vi "Fluke Molbox 1 Plus Acquire Totalize Cycle Results.vi"(0 "VISA resource name":refnum<visa-resource-name>, 1 "Gas Type (Nitrogen)":u16(ring) items=["Nitrogen", "Helium", "Argon", "Hydrogen", "Oxygen", "Methane", "Ethylene", "Propane", "Ethane", "Butane", "Carbon Monoxide", "Air", "Hexafluoroethane", "Nitrous Oxide", "Carbon Tetrafluoride", "Sulfur Hexafluoride", "Fluoroform", "Carbon Dioxide", "Xenon", "Octofluorocyclobutane"], 5 "Period Hours (0)":i32, 7 "Period Minutes (1)":i32=1, 9 "Period Seconds (0)":i32, 12 "K Factor (1.0)":dbl=1.0) -> (6 "Seconds Elapsed":dbl, 8 "Total Flow":dbl)   [LabVIEW 2023]
doc: "Completes a totalize cycle and returns the total flow that was accumulated in the cycle of which the length is inputted by the user."
uses:
  Fluke Molbox 1 Plus.lvlib
panel:
  in  "Serial Configuration":T1={"Baud Rate"=9600, "Parity"=0, "Data Bits"=7, "Stop Bits"=10} {"Stop Bits" items=["1"=10, "2"=20]; "Data Bits" items=["7"=7, "8"=8]; "Parity" items=["None", "Odd", "Even"]; "Baud Rate" items=["300"=300, "600"=600, "1200"=1200, "2400"=2400, "4800"=4800, "9600"=9600, "19200"=19200]}
  # "(c) 2012 National Instruments.  ALL RIGHTS RESERVED."
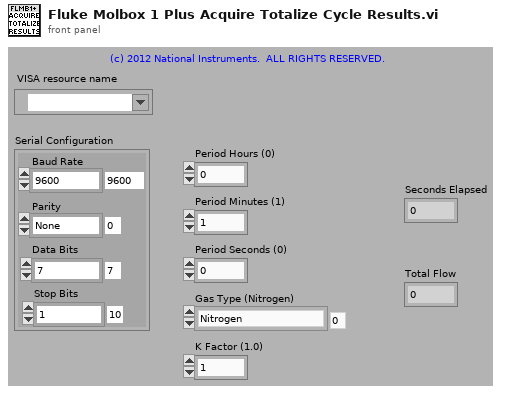
[diagram p1: front panel]
types:
  T1 = cluster{"Baud Rate":u32, "Parity":u16, "Data Bits":u16, "Stop Bits":u16}
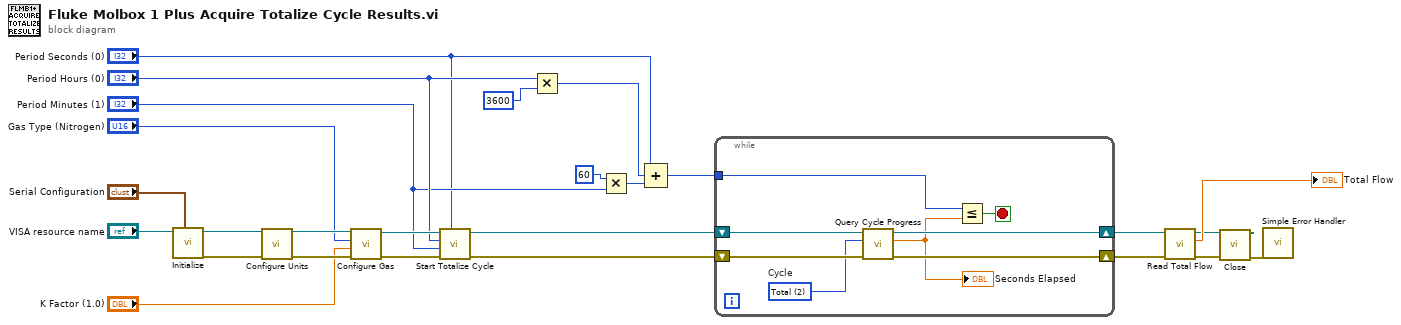
[diagram p0: block diagram]
diagram:
  n1 = call "Initialize.vi"("Serial Configuration"="Serial Configuration", "VISA resource name"="VISA resource name") -> ("error out"=w24:errorcluster, "VISA resource name out"=w25:refnum<visa-resource-name>)  [unwired: 8 in]
  n2 = call "Configure Units.vi"("VISA resource name"=w25, "error in (no error)"=w24) -> ("VISA resource name out"=w21:refnum<visa-resource-name>, "error out"=w20:errorcluster)  [unwired: 12 in]
  n3 = call "Configure Gas.vi"("error in (no error)"=w20, "K Factor (1.0)"="K Factor (1.0)", "Gas Type (0: Nitrogen)"="Gas Type (Nitrogen)", "VISA resource name"=w21) -> ("error out"=w14:errorcluster, "VISA resource name out"=w15:refnum<visa-resource-name>)  [unwired: 6 in]
  n4 = call "Start Totalize Cycle.vi"("Period Seconds (0)"="Period Seconds (0)", "error in (no error)"=w14, "Period Minutes (1)"="Period Minutes (1)", "Period Hours (0)"="Period Hours (0)", "VISA resource name"=w15) -> ("error out"=w16:errorcluster, "VISA resource name out"=w17:refnum<visa-resource-name>)  [unwired: 5 in]
  n5 = Multiply(x="Period Hours (0)", y=u32 3600) -> (x*y=w7:u32)
  n6 = Multiply(x=u32 60, y="Period Minutes (1)") -> (x*y=w8:u32)
  n7 = Compound Arithmetic op=ADD("Period Seconds (0)", w7, w8) -> (w5:u32)
  n8 = while {
    shift-right: [w29] -> w22
    shift-left: w16 -> [w33]
    shift-right: [w30] -> w23
    shift-left: w17 -> [w34]
    tunnel: w5 -> [w28]
    stop <- w32 stop-if-true
    w31 = u16 2 items=["Leak Check", "Purge", "Total"]  # Cycle
    n9 = call "Query Cycle Progress.vi"("error in (no error)"=w33, "Cycle (0: Average Flow)"=w31, "VISA resource name"=w34) -> ("error out"=w29:errorcluster, "Seconds"=w27:dbl, "VISA resource name out"=w30:refnum<visa-resource-name>)  [unwired: 6 in]
    "Seconds Elapsed" <- w27
    n10 = Less Or Equal?(x=w28, y=w27) -> (x <= y?=w32:bool)
  }
  n11 = call "Read Total Flow.vi"("error in (no error)"=w22, "VISA resource name"=w23) -> ("error out"=w2:errorcluster, "Total Flow"=→"Total Flow":dbl, "VISA resource name out"=w3:refnum<visa-resource-name>)  [unwired: 7 in]
  n12 = call "Close.vi"("error in (no error)"=w2, "VISA resource name"=w3) -> ("error out"=w4:errorcluster)  [unwired: 9 in]
  n13 = call <vilib>:"Simple Error Handler.vi"("error in (no error)"=w4) -> ()  [unwired: 4 in, 5 out]
